vi "SCMP - Build Recipe Paths.vi"(0 "Start path":path, 1 "Selected Cookbook":path) -> (5 "Cookbook * Comments":string, 7 "Recipe Not Found":bool[](array[boolean]), 8 "List of Recipes":path[](array[path]), 10 "error out":errorcluster)   [LabVIEW 2014]
doc: "Use this template to build a VI to use as a subVI."
panel:
  in  "stop":bool
  out "Output":string
  out "# of Recipes":i32
  out "Cookbook % Comments":string="*This is a test comment\r\n*test comment 2\r\n* test comment 3"
  out "\\basic Folders":path[](array[path])
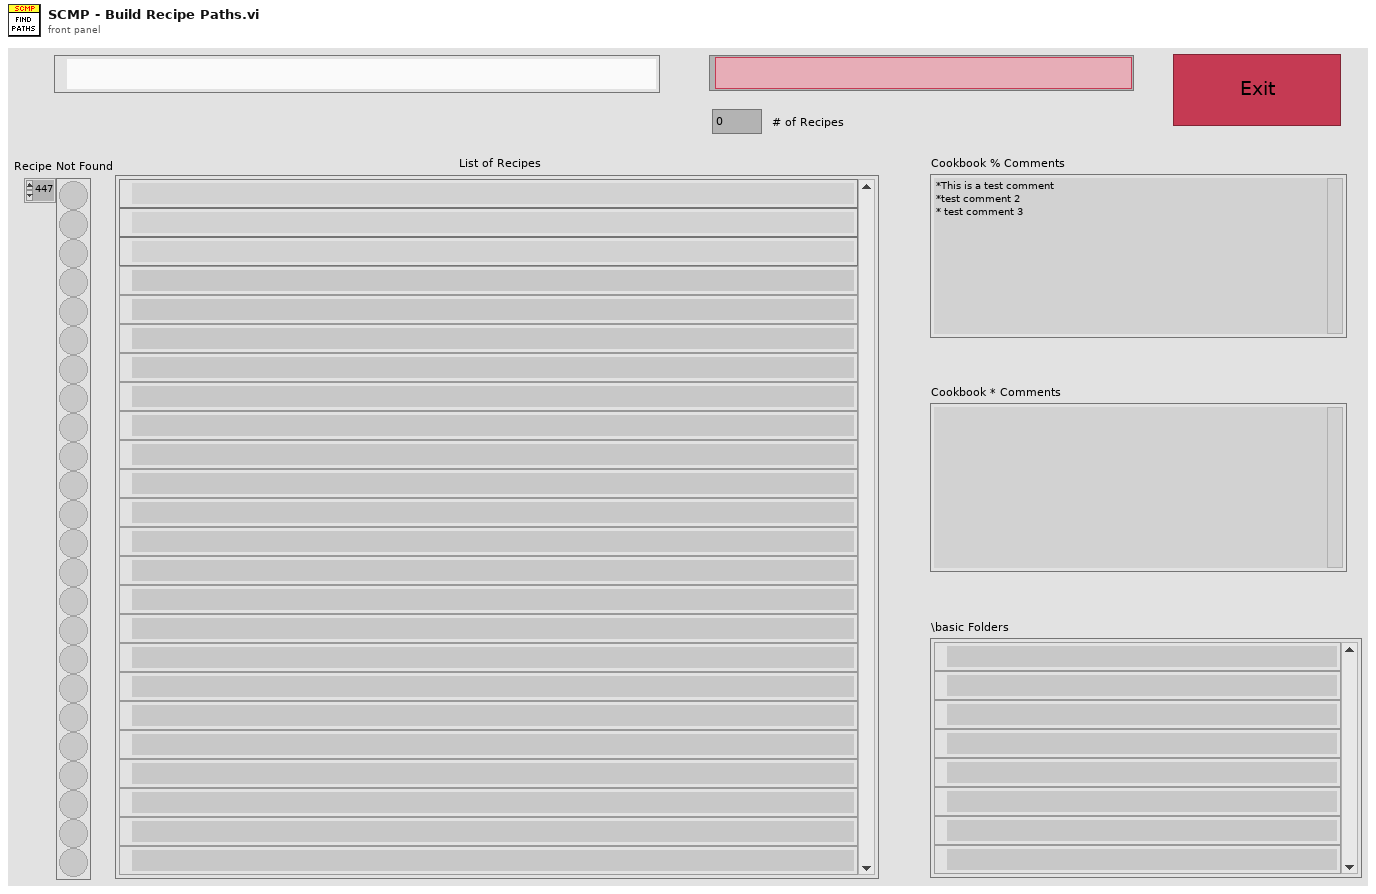
[diagram p1: front panel]
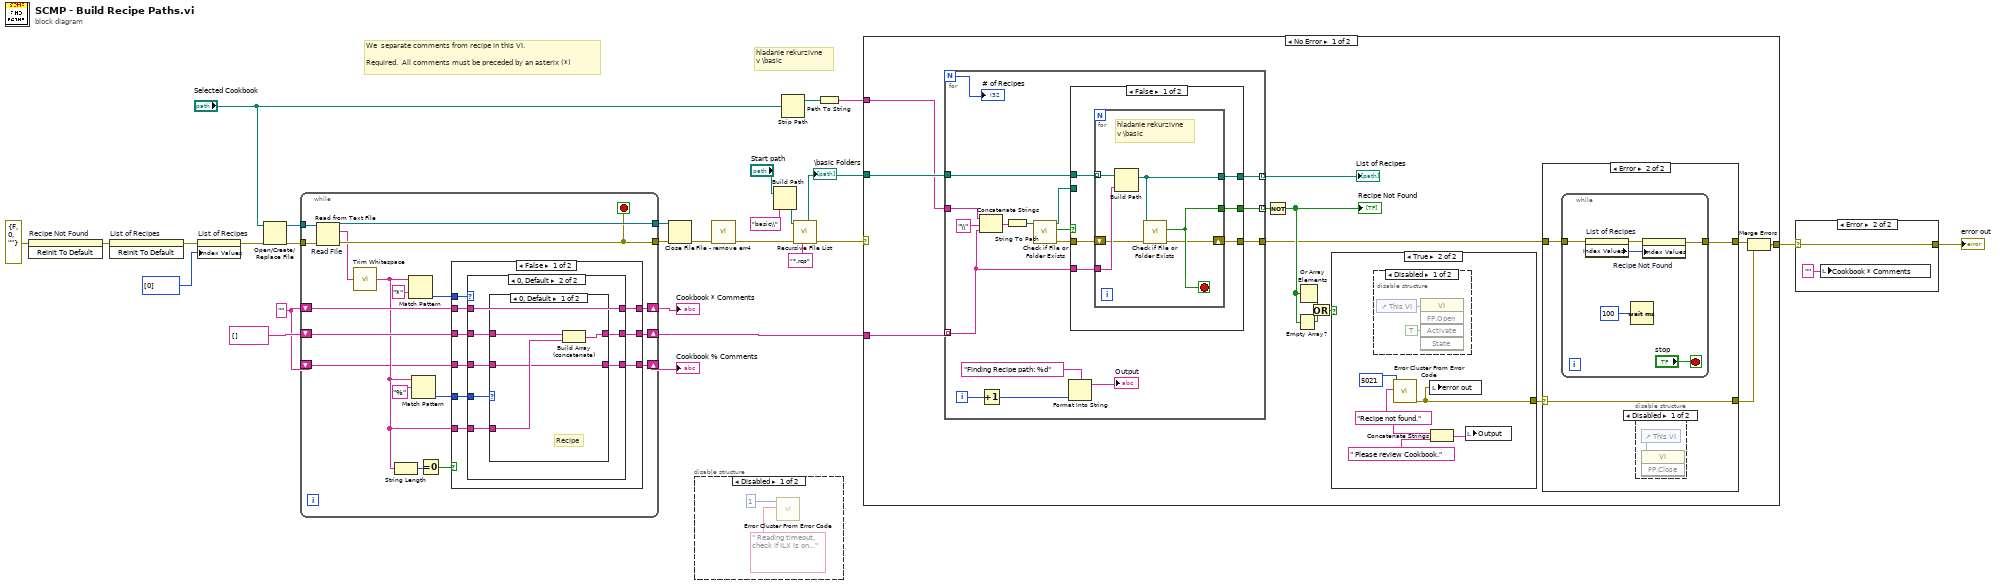
[diagram p0: block diagram]
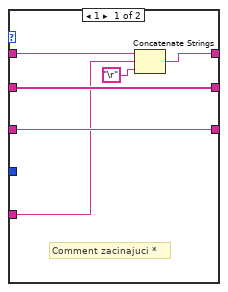
[diagram p10: hidden frame]
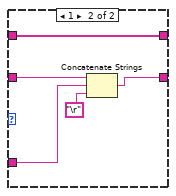
[diagram p11: hidden frame]
diagram:
  w14 = "" ("regular expression")
  # "hladanie rekurzivne\nv \\basic"
  # "We  separate comments from recipe in this VI.\n\nRequired.  All comments must be preceded by an asterix (*)"
  n1 = invoke on="Recipe Not Found" class="Arr (strict)" method="Reinit To Default"(error in=errorcluster {"status"=FALSE, "code"=0, "source"=""} ("error in (no error)")) -> (error out=w7:errorcluster)  [unwired: 2 in, 2 out]
  n2 = invoke on="List of Recipes" class="Arr (strict)" method="Reinit To Default"(error in=w7) -> (error out=w6:errorcluster)  [unwired: 2 in, 2 out]
  n3 = property on="List of Recipes" class="Arr (strict)"(error in=w6, "Index Values"=u32[] [0]) -> (error out=w5:errorcluster)  [unwired: 1 in, 1 out]
  n4 = Open/Create/Replace File(file path (use dialog)="Selected Cookbook", error in=w5) -> (refnum out=w27:refnum<file>, error out=w26:errorcluster)  [unwired: 4 in, 1 out]
  n5 = while {
    tunnel: w27 -> [w45]
    tunnel: w26 -> [w44]
    shift-right: [w41] -> w25
    shift-left: w14 -> [w42]
    shift-right: [w28] -> w15
    shift-left: string[] [] ("array of recipes") -> [w40]
    tunnel: [w39] -> w23
    tunnel: [w38] -> w22
    shift-right: [w29] -> w13
    shift-left: w14 -> [w30]
    stop <- w38 stop-if-true
    n6 = Read from Text File "Read File"(file (use dialog)=w45, error in=w44) -> (refnum out=w39:refnum<file>, text=w34:string, error out=w38:errorcluster)  [unwired: 3 out]
    n7 = call <vilib>:"Trim Whitespace.vi"("string"=w34) -> ("trimmed string"=w33:string)  [unwired: 1 in]
    n8 = String Length(string=w33) -> (length=w36:i32)
    n9 = Match Pattern(string=w33, regular expression="*") -> (offset past match=w37:i32)  [unwired: 1 in, 3 out]
    n10 = Match Pattern(string=w33, regular expression="%") -> (offset past match=w31:i32)  [unwired: 1 in, 3 out]
    n11 = Equal To 0?(x=w36) -> (x = 0?=w35:bool)
    n12 = case shown="False" w35 {
      tunnel: w42 -> [w54 w79]
      tunnel: [w53 w79] -> w41
      tunnel: w40 -> [w52 w78]
      tunnel: [w51 w78] -> w28
      tunnel: w37 -> [w50 _]
      tunnel: w33 -> [w49 _]
      tunnel: w31 -> [w48 _]
      tunnel: w30 -> [w47 w77]
      tunnel: [w46 w77] -> w29
      frame False {
        n13 = case shown="0, Default" w50 {
          tunnel: w54 -> [w59 w67]
          tunnel: [w60 w67] -> w53
          tunnel: w49 -> [w56 w64]
          tunnel: w52 -> [w58 w66]
          tunnel: [w58 w65] -> w51
          tunnel: w48 -> [_ w63]
          tunnel: w47 -> [w57 w62]
          tunnel: [w57 w61] -> w46
          frame 1 {
            # "Comment zacinajuci *"
            n14 = Concatenate Strings(w59, w56, "\r") -> (w60:string)
          }
          frame 0, Default {
            n15 = case shown="0, Default" w63 {
              tunnel: w66 -> [w71 w74]
              tunnel: [w70 w74] -> w65
              tunnel: w64 -> [w69 w73]
              tunnel: w62 -> [w68 w76]
              tunnel: [w68 w75] -> w61
              frame 0, Default {
                # "Recipe"
                n16 = Build Array (concatenate)(w71, w69) -> (w70:string[])
              }
              frame 1 {
                n17 = Concatenate Strings(w76, w73, "\r") -> (w75:string)
              }
            }
          }
        }
      }
      frame True {
        # "prazdne riadky"
      }
    }
  }
  "Cookbook * Comments" <- w25
  "Cookbook % Comments" <- w13
  n18 = Close File(refnum=w23, error in=w22) -> (error out=w12:errorcluster)  [unwired: 1 out]
  n19 = disable-structure shown="Disabled" {
    frame Disabled {
      n20 = call <vilib>:"Error Cluster From Error Code.vi"("error message (\"\")"=" Reading timeout, check if ILX is on..." ("error message (\"\")"), "error code (0)"=1) -> ()  [unwired: 7 in, 1 out]
    }
    frame Enabled {
    }
  }
  n21 = call "File - remove err4.vi"("error in (no error)"=w12) -> ("error out"=w11:errorcluster)  [unwired: 10 in]
  n22 = Build Path(base path="Start path", name or relative path="basic\\" ("string")) -> (appended path=w20:path)
  n23 = Strip Path(path="Selected Cookbook") -> (stripped path=w3:path)  [unwired: 1 out]
  n24 = call <vilib>:"Recursive File List.vi"("pattern"="*.rcp", "error in (no error)"=w11, "Folder Path"=w20) -> ("error out"=w16:errorcluster, "All Folders"=w17:path[])  [unwired: 4 in, 3 out]
  "\\basic Folders" <- w17
  n25 = Path To String(path=w3) -> (string=w2:string)
  n26 = case shown="No Error" w16 {
    selector: w16 -> [_ w146]
    tunnel: w15 -> [w95 _]
    tunnel: w17 -> [w94 _]
    tunnel: [w85 w146] -> w10
    tunnel: w2 -> [w82 _]
    frame No Error {
      n27 = for {
        N -> [w119]
        tunnel: w95 -> [w122] mode=indexing
        tunnel: [w123] -> w90 mode=indexing
        tunnel: [w126] -> w91 mode=indexing
        tunnel: w82 -> [w125]
        tunnel: w94 -> [w124]
        tunnel: [w120] -> w84
        i -> [w118]
        n28 = Concatenate Strings(w125, "\\" ("string"), w122) -> (w129:string)
        n29 = Increment(x=w118) -> (x+1=w116:i32)
        n30 = String To Path(string=w129) -> (path=w127:path)
        n31 = call <vilib>:"Check if File or Folder Exists.vi"("path"=w127) -> ("error out"=w121:errorcluster, "file or folder exists?"=w128:bool)  [unwired: 8 in, 1 out]
        n32 = Format Into String(format string="Finding Recipe path: %d", w116) -> (resulting string=→"Output":string)  [unwired: 2 in, 1 out]
        n33 = case shown="False" w128 {
          selector: w128 -> [_ w145]
          tunnel: [w136 w145] -> w123
          tunnel: w127 -> [_ w144]
          tunnel: [w135 w144] -> w126
          tunnel: w124 -> [w134 _]
          tunnel: w122 -> [w133 _]
          tunnel: w121 -> [w131 w143]
          tunnel: [w132 w143] -> w120
          frame False {
            n34 = for {
              tunnel: [w139] -> w136
              tunnel: w133 -> [w142]
              tunnel: [w141] -> w135
              tunnel: w134 -> [w140] mode=indexing
              shift-right: [w138] -> w132
              shift-left: w131 -> [w137]
              stop <- w139 stop-if-true
              # "hladanie rekurzivne\nv \\basic"
              n35 = Build Path(base path=w140, name or relative path=w142) -> (appended path=w141:path)
              n36 = call <vilib>:"Check if File or Folder Exists.vi"("error in (no error)"=w137, "path"=w141) -> ("error out"=w138:errorcluster, "file or folder exists?"=w139:bool)  [unwired: 7 in, 1 out]
            }
          }
          frame True {
          }
        }
        "# of Recipes" <- w119
      }
      "List of Recipes" <- w91
      n37 = Not(x=w90) -> (.not. x?=w88:bool[])
      "Recipe Not Found" <- w88
      n38 = Empty Array?(array=w88) -> (empty?=w93:bool)
      n39 = Or Array Elements(Boolean array=w88) -> (logical OR=w89:bool)
      n40 = Or(x=w89, y=w93) -> (x .or. y?=w92:bool)
      n41 = case shown="True" w92 {
        tunnel: [_ w111] -> w87
        frame False {
        }
        frame True {
          w110 = "Recipe not found." ("message")
          n42 = disable-structure shown="Disabled" {
            frame Disabled {
              n43 = control-ref of="This VI"() -> (w113:refnum<vi>)
              n44 = invoke class="VI" method="FP.Open"(reference=w113, "Activate"=TRUE ("Activate?")) -> ()  [unwired: 3 in, 5 out]
            }
            frame Enabled {
            }
          }
          n45 = call <vilib>:"Error Cluster From Error Code.vi"("error message (\"\")"=w110, "error code (0)"=5021) -> ("error out"=w111:errorcluster)  [unwired: 7 in]
          n46 = local write "error out"(w111) -> ()
          n47 = Concatenate Strings(w110, " Please review Cookbook." ("message")) -> (w108:string)
          n48 = local write "Output"(w108) -> ()
        }
      }
      n49 = case shown="Error" w87 {
        selector: w87 -> [w97 w100]
        tunnel: [w97 w100] -> w86
        tunnel: w84 -> [w96 w99]
        tunnel: [w96 w98] -> w83
        frame No Error {
        }
        frame Error {
          n50 = while {
            tunnel: w99 -> [w103]
            tunnel: [w101] -> w98
            stop <- "stop" stop-if-true
            n51 = property on="List of Recipes" class="Arr (strict)"(error in=w103) -> (error out=w102:errorcluster, "Index Values"=w104:u32[])  [unwired: 1 in, 1 out]
            n52 = Wait (ms)(milliseconds to wait=u32 100) -> ()  [unwired: 1 out]
            n53 = property on="Recipe Not Found" class="Arr (strict)"(error in=w102, "Index Values"=w104) -> (error out=w101:errorcluster)  [unwired: 1 in, 1 out]
          }
          n54 = disable-structure shown="Disabled" {
            frame Disabled {
              n55 = control-ref of="This VI"() -> (w107:refnum<vi>)
              n56 = invoke class="VI" method="FP.Close"(reference=w107) -> ()  [unwired: 2 in, 3 out]
            }
            frame Enabled {
            }
          }
        }
      }
      n57 = Merge Errors(w83, w86) -> (w85:errorcluster)
    }
    frame Error {
    }
  }
  n58 = case shown="Error" w10 {
    selector: w10 -> [w147 w148]
    tunnel: [w147 w148] -> w9
    frame No Error {
    }
    frame Error {
      n59 = local write "Cookbook * Comments"("" ("Cookbook * Comments")) -> ()
    }
  }
  "error out" <- w9
